vi "New Report Line.vi"(0 "report in":refnum<class "NI_Standard Report.lvclass">, 9 "number of lines (1)":i32=1, 11 "error in (no error)":errorcluster) -> (4 "report out":refnum<class "NI_Standard Report.lvclass">, 15 "error out":errorcluster)   [LabVIEW 2015, in "NI_Standard Report.lvclass"]
doc: "Starts a new line in the report."
uses:
  <vilib>/Utility/NIReport.llb/Standard Report/NI_Standard Report.lvclass
  <vilib>/Utility/NIReport.llb/Standard Report/NI_Standard Report.lvclass/NI_Standard Report.ctl
  <vilib>/Utility/NIReport.llb/NI_ReportGenerationCore.lvlib
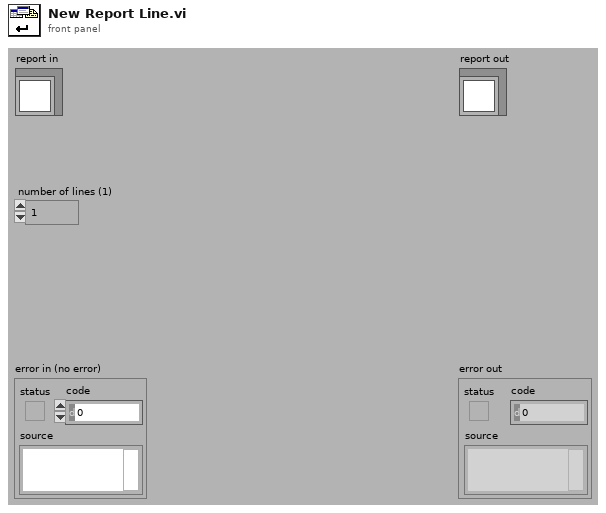
[diagram p1: front panel]
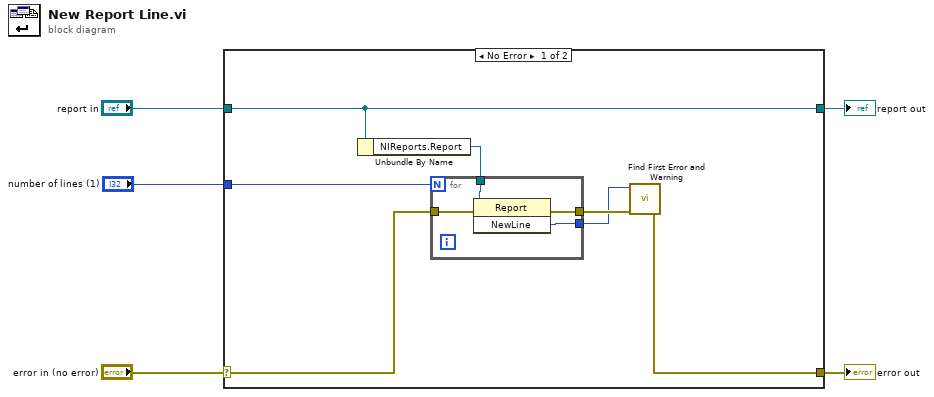
[diagram p0: block diagram]
diagram:
  n1 = case shown="No Error" "error in (no error)" {
    selector: "error in (no error)" -> [w8 w18]
    tunnel: [w7 w18] -> w4
    tunnel: [w6 w17] -> w2
    tunnel: "report in" -> [w6 w17]
    tunnel: "number of lines (1)" -> [w9 _]
    frame No Error {
      n2 = Unbundle By Name(w6) -> ("NIReports.Report"=w12:refnum<k7>)
      n3 = for {
        N: w9 -> [_]
        tunnel: w8 -> [w16]
        tunnel: [w15] -> w10
        tunnel: [w14] -> w11
        tunnel: w12 -> [w13]
        n4 = invoke on="Invoke Node" class="Report" method="NewLine"(reference=w13, error in=w16) -> (error out=w14:errorcluster, "NewLine"=w15:i32)  [unwired: 1 in, 1 out]
      }
      n5 = call <vilib>:"Find First Error and Warning.vi"("error in (no error)"=w11, "error code"=w10) -> ("error out"=w7:errorcluster)  [unwired: 1 in, 4 out]
    }
    frame Error {
    }
  }
  "error out" <- w4
  "report out" <- w2
